vi "monitor -- write section files.vi"(4 "Magn Field (T)":dbl, 6 "temperature":dbl, 10 "Sweep folder path":path=path "C:/Data/GloveBox/Pu-delta-2-20120625/sweep2", 11 "Array":T1[](array[typedef])=[{"delta"=0.0, "gamma"=0.0, "exp"=0.0, "found?"=FALSE, "found"=0.0, "gamma found"=0.0, "init linear"=FALSE, "interpolate"=enum."force", "gamma-factor"=3.5, "slope"=0.0, "update freq?"=FALSE, "update gamma?"=FALSE, "acc factor"=3.5, "linear interpolation state"={"requested size"=20, "Array"=[], "actual number of elements"=0}, "ind"=0.0, "gamma ratio"=0.0, "gamma off limit?"=FALSE, "freq off limit?"=FALSE}, {"delta"=0.0, "gamma"=0.0, "exp"=0.0, "found?"=FALSE, "found"=0.0, "gamma found"=0.0, "init linear"=FALSE, "interpolate"=enum."force", "gamma-factor"=3.5, "slope"=0.0, "update freq?"=FALSE, "update gamma?"=FALSE, "acc factor"=3.5, "linear interpolation state"={"requested size"=20, "Array"=[], "actual number of elements"=0}, "ind"=0.0, "gamma ratio"=0.0, "gamma off limit?"=FALSE, "freq off limit?"=FALSE}, {"delta"=0.0, "gamma"=0.0, "exp"=0.0, "found?"=FALSE, "found"=0.0, "gamma found"=0.0, "init linear"=FALSE, "interpolate"=enum."force", "gamma-factor"=3.5, "slope"=0.0, "update freq?"=FALSE, "update gamma?"=FALSE, "acc factor"=3.5, "linear interpolation state"={"requested size"=20, "Array"=[], "actual number of elements"=0}, "ind"=0.0, "gamma ratio"=0.0, "gamma off limit?"=FALSE, "freq off limit?"=FALSE}, {"delta"=0.0, "gamma"=0.0, "exp"=0.0, "found?"=FALSE, "found"=0.0, "gamma found"=0.0, "init linear"=FALSE, "interpolate"=enum."force", "gamma-factor"=3.5, "slope"=0.0, "update freq?"=FALSE, "update gamma?"=FALSE, "acc factor"=3.5, "linear interpolation state"={"requested size"=20, "Array"=[], "actual number of elements"=0}, "ind"=0.0, "gamma ratio"=0.0, "gamma off limit?"=FALSE, "freq off limit?"=FALSE}, {"delta"=0.0, "gamma"=0.0, "exp"=0.0, "found?"=FALSE, "found"=0.0, "gamma found"=0.0, "init linear"=FALSE, "interpolate"=enum."force", "gamma-factor"=3.5, "slope"=0.0, "update freq?"=FALSE, "update gamma?"=FALSE, "acc factor"=3.5, "linear interpolation state"={"requested size"=20, "Array"=[], "actual number of elements"=0}, "ind"=0.0, "gamma ratio"=0.0, "gamma off limit?"=FALSE, "freq off limit?"=FALSE}, {"delta"=0.0, "gamma"=0.0, "exp"=0.0, "found?"=FALSE, "found"=0.0, "gamma found"=0.0, "init linear"=FALSE, "interpolate"=enum."force", "gamma-factor"=3.5, "slope"=0.0, "update freq?"=FALSE, "update gamma?"=FALSE, "acc factor"=3.5, "linear interpolation state"={"requested size"=20, "Array"=[], "actual number of elements"=0}, "ind"=0.0, "gamma ratio"=0.0, "gamma off limit?"=FALSE, "freq off limit?"=FALSE}, {"delta"=0.0, "gamma"=0.0, "exp"=0.0, "found?"=FALSE, "found"=0.0, "gamma found"=0.0, "init linear"=FALSE, "interpolate"=enum."force", "gamma-factor"=3.5, "slope"=0.0, "update freq?"=FALSE, "update gamma?"=FALSE, "acc factor"=3.5, "linear interpolation state"={"requested size"=20, "Array"=[], "actual number of elements"=0}, "ind"=0.0, "gamma ratio"=0.0, "gamma off limit?"=FALSE, "freq off limit?"=FALSE}, {"delta"=0.0, "gamma"=0.0, "exp"=0.0, "found?"=FALSE, "found"=0.0, "gamma found"=0.0, "init linear"=FALSE, "interpolate"=enum."force", "gamma-factor"=3.5, "slope"=0.0, "update freq?"=FALSE, "update gamma?"=FALSE, "acc factor"=3.5, "linear interpolation state"={"requested size"=20, "Array"=[], "actual number of elements"=0}, "ind"=0.0, "gamma ratio"=0.0, "gamma off limit?"=FALSE, "freq off limit?"=FALSE}, {"delta"=0.0, "gamma"=0.0, "exp"=0.0, "found?"=FALSE, "found"=0.0, "gamma found"=0.0, "init linear"=FALSE, "interpolate"=enum."force", "gamma-factor"=3.5, "slope"=0.0, "update freq?"=FALSE, "update gamma?"=FALSE, "acc factor"=3.5, "linear interpolation state"={"requested size"=20, "Array"=[], "actual number of elements"=0}, "ind"=0.0, "gamma ratio"=0.0, "gamma off limit?"=FALSE, "freq off limit?"=FALSE}, {"delta"=0.0, "gamma"=0.0, "exp"=0.0, "found?"=FALSE, "found"=0.0, "gamma found"=0.0, "init linear"=FALSE, "interpolate"=enum."force", "gamma-factor"=3.5, "slope"=0.0, "update freq?"=FALSE, "update gamma?"=FALSE, "acc factor"=3.5, "linear interpolation state"={"requested size"=20, "Array"=[], "actual number of elements"=0}, "ind"=0.0, "gamma ratio"=0.0, "gamma off limit?"=FALSE, "freq off limit?"=FALSE}, {"delta"=0.0, "gamma"=0.0, "exp"=0.0, "found?"=FALSE, "found"=0.0, "gamma found"=0.0, "init linear"=FALSE, "interpolate"=enum."force", "gamma-factor"=3.5, "slope"=0.0, "update freq?"=FALSE, "update gamma?"=FALSE, "acc factor"=3.5, "linear interpolation state"={"requested size"=20, "Array"=[], "actual number of elements"=0}, "ind"=0.0, "gamma ratio"=0.0, "gamma off limit?"=FALSE, "freq off limit?"=FALSE}, {"delta"=0.0, "gamma"=0.0, "exp"=0.0, "found?"=FALSE, "found"=0.0, "gamma found"=0.0, "init linear"=FALSE, "interpolate"=enum."force", "gamma-factor"=3.5, "slope"=0.0, "update freq?"=FALSE, "update gamma?"=FALSE, "acc factor"=3.5, "linear interpolation state"={"requested size"=20, "Array"=[], "actual number of elements"=0}, "ind"=0.0, "gamma ratio"=0.0, "gamma off limit?"=FALSE, "freq off limit?"=FALSE}, {"delta"=0.0, "gamma"=0.0, "exp"=0.0, "found?"=FALSE, "found"=0.0, "gamma found"=0.0, "init linear"=FALSE, "interpolate"=enum."force", "gamma-factor"=3.5, "slope"=0.0, "update freq?"=FALSE, "update gamma?"=FALSE, "acc factor"=3.5, "linear interpolation state"={"requested size"=20, "Array"=[], "actual number of elements"=0}, "ind"=0.0, "gamma ratio"=0.0, "gamma off limit?"=FALSE, "freq off limit?"=FALSE}, {"delta"=0.0, "gamma"=0.0, "exp"=0.0, "found?"=FALSE, "found"=0.0, "gamma found"=0.0, "init linear"=FALSE, "interpolate"=enum."force", "gamma-factor"=3.5, "slope"=0.0, "update freq?"=FALSE, "update gamma?"=FALSE, "acc factor"=3.5, "linear interpolation state"={"requested size"=20, "Array"=[], "actual number of elements"=0}, "ind"=0.0, "gamma ratio"=0.0, "gamma off limit?"=FALSE, "freq off limit?"=FALSE}, {"delta"=0.0, "gamma"=0.0, "exp"=0.0, "found?"=FALSE, "found"=0.0, "gamma found"=0.0, "init linear"=FALSE, "interpolate"=enum."force", "gamma-factor"=3.5, "slope"=0.0, "update freq?"=FALSE, "update gamma?"=FALSE, "acc factor"=3.5, "linear interpolation state"={"requested size"=20, "Array"=[], "actual number of elements"=0}, "ind"=0.0, "gamma ratio"=0.0, "gamma off limit?"=FALSE, "freq off limit?"=FALSE}, {"delta"=0.0, "gamma"=0.0, "exp"=0.0, "found?"=FALSE, "found"=0.0, "gamma found"=0.0, "init linear"=FALSE, "interpolate"=enum."force", "gamma-factor"=3.5, "slope"=0.0, "update freq?"=FALSE, "update gamma?"=FALSE, "acc factor"=3.5, "linear interpolation state"={"requested size"=20, "Array"=[], "actual number of elements"=0}, "ind"=0.0, "gamma ratio"=0.0, "gamma off limit?"=FALSE, "freq off limit?"=FALSE}, {"delta"=0.0, "gamma"=0.0, "exp"=0.0, "found?"=FALSE, "found"=0.0, "gamma found"=0.0, "init linear"=FALSE, "interpolate"=enum."force", "gamma-factor"=3.5, "slope"=0.0, "update freq?"=FALSE, "update gamma?"=FALSE, "acc factor"=3.5, "linear interpolation state"={"requested size"=20, "Array"=[], "actual number of elements"=0}, "ind"=0.0, "gamma ratio"=0.0, "gamma off limit?"=FALSE, "freq off limit?"=FALSE}, {"delta"=0.0, "gamma"=0.0, "exp"=0.0, "found?"=FALSE, "found"=0.0, "gamma found"=0.0, "init linear"=FALSE, "interpolate"=enum."force", "gamma-factor"=3.5, "slope"=0.0, "update freq?"=FALSE, "update gamma?"=FALSE, "acc factor"=3.5, "linear interpolation state"={"requested size"=20, "Array"=[], "actual number of elements"=0}, "ind"=0.0, "gamma ratio"=0.0, "gamma off limit?"=FALSE, "freq off limit?"=FALSE}, {"delta"=0.0, "gamma"=0.0, "exp"=0.0, "found?"=FALSE, "found"=0.0, "gamma found"=0.0, "init linear"=FALSE, "interpolate"=enum."force", "gamma-factor"=3.5, "slope"=0.0, "update freq?"=FALSE, "update gamma?"=FALSE, "acc factor"=3.5, "linear interpolation state"={"requested size"=20, "Array"=[], "actual number of elements"=0}, "ind"=0.0, "gamma ratio"=0.0, "gamma off limit?"=FALSE, "freq off limit?"=FALSE}, {"delta"=0.0, "gamma"=0.0, "exp"=0.0, "found?"=FALSE, "found"=0.0, "gamma found"=0.0, "init linear"=FALSE, "interpolate"=enum."force", "gamma-factor"=3.5, "slope"=0.0, "update freq?"=FALSE, "update gamma?"=FALSE, "acc factor"=3.5, "linear interpolation state"={"requested size"=20, "Array"=[], "actual number of elements"=0}, "ind"=0.0, "gamma ratio"=0.0, "gamma off limit?"=FALSE, "freq off limit?"=FALSE}, {"delta"=0.0, "gamma"=0.0, "exp"=0.0, "found?"=FALSE, "found"=0.0, "gamma found"=0.0, "init linear"=FALSE, "interpolate"=enum."force", "gamma-factor"=3.5, "slope"=0.0, "update freq?"=FALSE, "update gamma?"=FALSE, "acc factor"=3.5, "linear interpolation state"={"requested size"=20, "Array"=[], "actual number of elements"=0}, "ind"=0.0, "gamma ratio"=0.0, "gamma off limit?"=FALSE, "freq off limit?"=FALSE}, {"delta"=0.0, "gamma"=0.0, "exp"=0.0, "found?"=FALSE, "found"=0.0, "gamma found"=0.0, "init linear"=FALSE, "interpolate"=enum."force", "gamma-factor"=3.5, "slope"=0.0, "update freq?"=FALSE, "update gamma?"=FALSE, "acc factor"=3.5, "linear interpolation state"={"requested size"=20, "Array"=[], "actual number of elements"=0}, "ind"=0.0, "gamma ratio"=0.0, "gamma off limit?"=FALSE, "freq off limit?"=FALSE}, {"delta"=0.0, "gamma"=0.0, "exp"=0.0, "found?"=FALSE, "found"=0.0, "gamma found"=0.0, "init linear"=FALSE, "interpolate"=enum."force", "gamma-factor"=3.5, "slope"=0.0, "update freq?"=FALSE, "update gamma?"=FALSE, "acc factor"=3.5, "linear interpolation state"={"requested size"=20, "Array"=[], "actual number of elements"=0}, "ind"=0.0, "gamma ratio"=0.0, "gamma off limit?"=FALSE, "freq off limit?"=FALSE}, {"delta"=0.0, "gamma"=0.0, "exp"=0.0, "found?"=FALSE, "found"=0.0, "gamma found"=0.0, "init linear"=FALSE, "interpolate"=enum."force", "gamma-factor"=3.5, "slope"=0.0, "update freq?"=FALSE, "update gamma?"=FALSE, "acc factor"=3.5, "linear interpolation state"={"requested size"=20, "Array"=[], "actual number of elements"=0}, "ind"=0.0, "gamma ratio"=0.0, "gamma off limit?"=FALSE, "freq off limit?"=FALSE}, {"delta"=0.0, "gamma"=0.0, "exp"=0.0, "found?"=FALSE, "found"=0.0, "gamma found"=0.0, "init linear"=FALSE, "interpolate"=enum."force", "gamma-factor"=3.5, "slope"=0.0, "update freq?"=FALSE, "update gamma?"=FALSE, "acc factor"=3.5, "linear interpolation state"={"requested size"=20, "Array"=[], "actual number of elements"=0}, "ind"=0.0, "gamma ratio"=0.0, "gamma off limit?"=FALSE, "freq off limit?"=FALSE}, {"delta"=0.0, "gamma"=0.0, "exp"=0.0, "found?"=FALSE, "found"=0.0, "gamma found"=0.0, "init linear"=FALSE, "interpolate"=enum."force", "gamma-factor"=3.5, "slope"=0.0, "update freq?"=FALSE, "update gamma?"=FALSE, "acc factor"=3.5, "linear interpolation state"={"requested size"=20, "Array"=[], "actual number of elements"=0}, "ind"=0.0, "gamma ratio"=0.0, "gamma off limit?"=FALSE, "freq off limit?"=FALSE}, {"delta"=0.0, "gamma"=0.0, "exp"=0.0, "found?"=FALSE, "found"=0.0, "gamma found"=0.0, "init linear"=FALSE, "interpolate"=enum."force", "gamma-factor"=3.5, "slope"=0.0, "update freq?"=FALSE, "update gamma?"=FALSE, "acc factor"=3.5, "linear interpolation state"={"requested size"=20, "Array"=[], "actual number of elements"=0}, "ind"=0.0, "gamma ratio"=0.0, "gamma off limit?"=FALSE, "freq off limit?"=FALSE}, {"delta"=0.0, "gamma"=0.0, "exp"=0.0, "found?"=FALSE, "found"=0.0, "gamma found"=0.0, "init linear"=FALSE, "interpolate"=enum."force", "gamma-factor"=3.5, "slope"=0.0, "update freq?"=FALSE, "update gamma?"=FALSE, "acc factor"=3.5, "linear interpolation state"={"requested size"=20, "Array"=[], "actual number of elements"=0}, "ind"=0.0, "gamma ratio"=0.0, "gamma off limit?"=FALSE, "freq off limit?"=FALSE}, {"delta"=0.0, "gamma"=0.0, "exp"=0.0, "found?"=FALSE, "found"=0.0, "gamma found"=0.0, "init linear"=FALSE, "interpolate"=enum."force", "gamma-factor"=3.5, "slope"=0.0, "update freq?"=FALSE, "update gamma?"=FALSE, "acc factor"=3.5, "linear interpolation state"={"requested size"=20, "Array"=[], "actual number of elements"=0}, "ind"=0.0, "gamma ratio"=0.0, "gamma off limit?"=FALSE, "freq off limit?"=FALSE}, {"delta"=0.0, "gamma"=0.0, "exp"=0.0, "found?"=FALSE, "found"=0.0, "gamma found"=0.0, "init linear"=FALSE, "interpolate"=enum."force", "gamma-factor"=3.5, "slope"=0.0, "update freq?"=FALSE, "update gamma?"=FALSE, "acc factor"=3.5, "linear interpolation state"={"requested size"=20, "Array"=[], "actual number of elements"=0}, "ind"=0.0, "gamma ratio"=0.0, "gamma off limit?"=FALSE, "freq off limit?"=FALSE}, {"delta"=0.0, "gamma"=0.0, "exp"=0.0, "found?"=FALSE, "found"=0.0, "gamma found"=0.0, "init linear"=FALSE, "interpolate"=enum."force", "gamma-factor"=3.5, "slope"=0.0, "update freq?"=FALSE, "update gamma?"=FALSE, "acc factor"=3.5, "linear interpolation state"={"requested size"=20, "Array"=[], "actual number of elements"=0}, "ind"=0.0, "gamma ratio"=0.0, "gamma off limit?"=FALSE, "freq off limit?"=FALSE}, {"delta"=0.0, "gamma"=0.0, "exp"=0.0, "found?"=FALSE, "found"=0.0, "gamma found"=0.0, "init linear"=FALSE, "interpolate"=enum."force", "gamma-factor"=3.5, "slope"=0.0, "update freq?"=FALSE, "update gamma?"=FALSE, "acc factor"=3.5, "linear interpolation state"={"requested size"=20, "Array"=[], "actual number of elements"=0}, "ind"=0.0, "gamma ratio"=0.0, "gamma off limit?"=FALSE, "freq off limit?"=FALSE}, {"delta"=0.0, "gamma"=0.0, "exp"=0.0, "found?"=FALSE, "found"=0.0, "gamma found"=0.0, "init linear"=FALSE, "interpolate"=enum."force", "gamma-factor"=3.5, "slope"=0.0, "update freq?"=FALSE, "update gamma?"=FALSE, "acc factor"=3.5, "linear interpolation state"={"requested size"=20, "Array"=[], "actual number of elements"=0}, "ind"=0.0, "gamma ratio"=0.0, "gamma off limit?"=FALSE, "freq off limit?"=FALSE}]) -> ()   [LabVIEW 2015]
uses:
  peak monitor ctl - V2.ctl
  interpolation state - real.ctl
  lorentzian.ctl
  circle corners.ctl
  ctl -- name dispatcher -- action.ctl
  next chunk read-write PID -- action.ctl
  file -- read-write control.ctl
  array -- find index - real.vi
  array -- interpolate -- i.vi
  Q -- check range -- i -- real.vi
  Q - not nan -- real.vi
  <vilib>/Utility/libraryn.llb/Check if File or Folder Exists.vi
  file -- read list of lines.vi
  parse -- find first line.vi
  parse -- get list of matches -- numbers.vi
  <vilib>/Utility/file.llb/Write To Spreadsheet File.vi
  <vilib>/Utility/file.llb/Write To Spreadsheet File (string).vi
  <vilib>/gmath/function.llb/Binomial Coefficient.vi
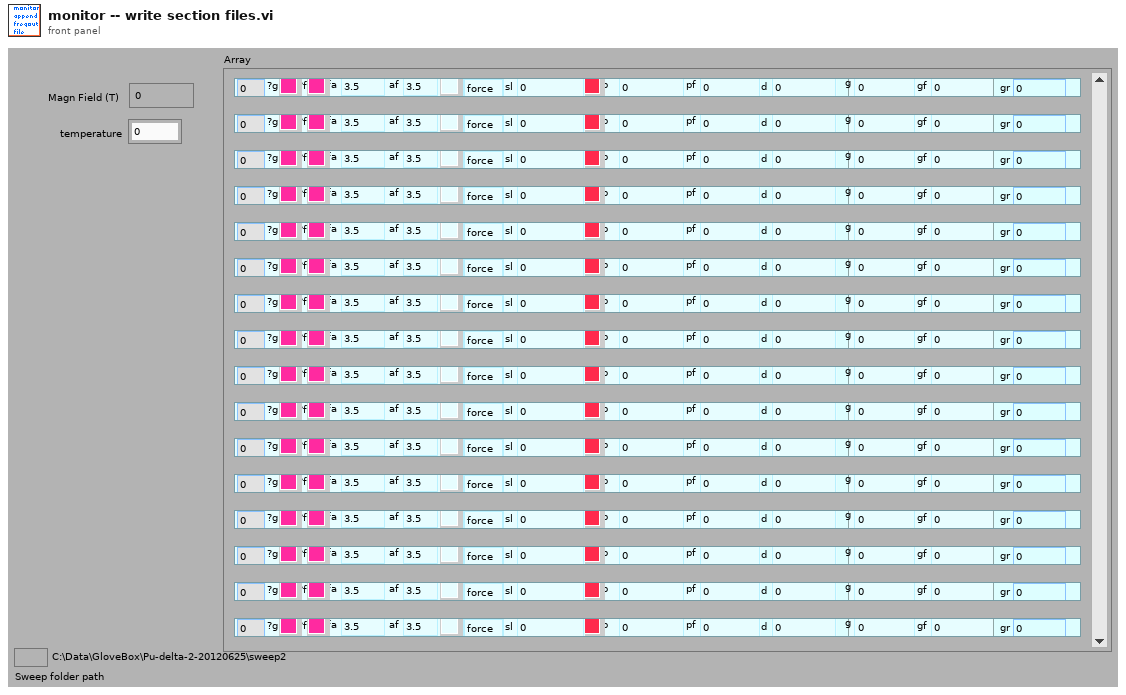
[diagram p1: front panel]
types:
  T1 = typedef "peak monitor ctl - V2.ctl" = cluster{"delta":dbl, "gamma":dbl, "exp":dbl, "found?":bool, "found":dbl, "gamma found":dbl, "init linear":bool, "interpolate":enum16{"line", "force"}, "gamma-factor":dbl, "slope":dbl, "update freq?":bool, "update gamma?":bool, "acc factor":dbl, "linear interpolation state":T2, "ind":dbl, "gamma ratio":dbl, "gamma off limit?":bool, "freq off limit?":bool}
  T2 = typedef "interpolation state - real.ctl" = cluster{"requested size":i32, "Array":dbl[], "actual number of elements":i32}
  T3 = typedef "ctl -- name dispatcher -- action.ctl" = enum16{"peak frequency", "peak frequency DUMP", "peak gamma DUMP", "peak gamma", "peak frequency TEST", "peak gamma TEST", "ultrasonic power", "time in gamma", "set temperature ", "set temperature timer", "peak default gamma", "last scan file", "peak freq gamma TEST", "peak NAMES", "errors", "P_I_D", "P", "I", "D", "power vs time", "power vs time TIMER", "void", "power log", "set temperature - SINE", "itc ltc log", "peak - time in gamma"}
  T4 = typedef "lorentzian.ctl" = cluster{"Amplitude":dbl, "omega(0)":dbl, "Gamma":dbl, "phase":dbl, "Q":dbl, "Norm  Ampl":dbl, "z (inf)":cdb, "4corners":T5}
  T5 = typedef "circle corners.ctl" = cluster{"z (-pi/2)":cdb, "z(inf)":cdb, "z (pi/2)":cdb, "z center":cdb, "z(0)":cdb, "radius":dbl}
  T6 = typedef "next chunk read-write PID -- action.ctl" = enum16{"read", "interpolate", "append col", "write", "write PID col", "append PID col", "interpolate - bezier"}
  T7 = typedef "file -- read-write control.ctl" = enum16{"read", "write all", "append one line"}
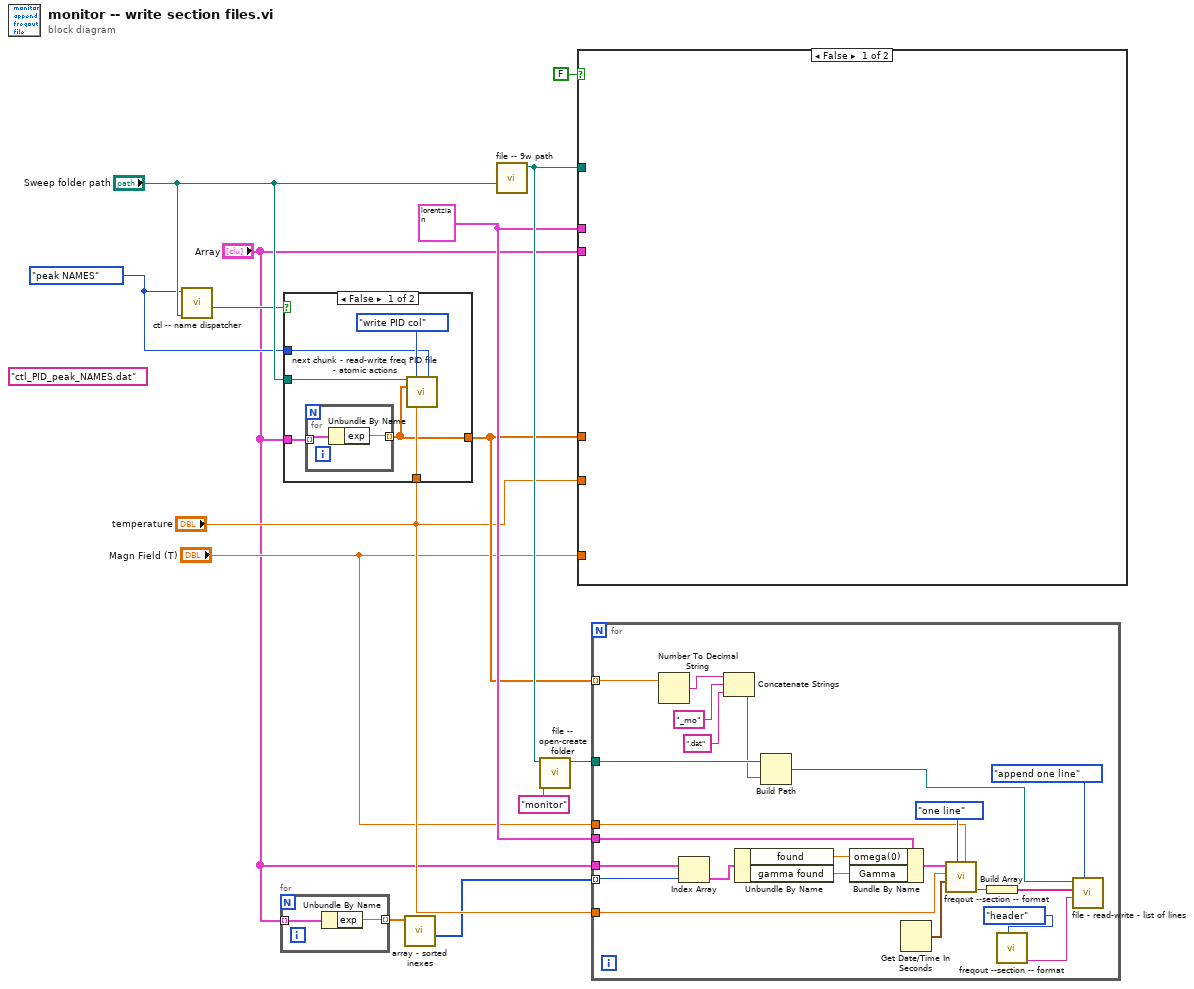
[diagram p0: block diagram]
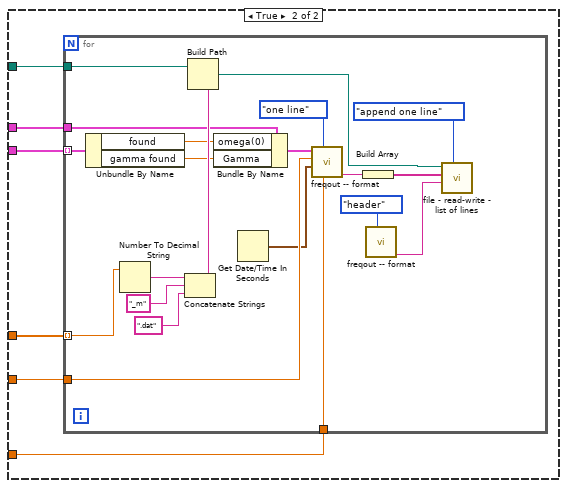
[diagram p2: hidden frame]
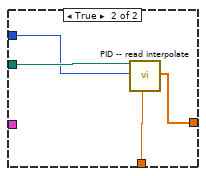
[diagram p3: hidden frame]
diagram:
  w6 = ctl_--_name_dispatcher_--_action."peak NAMES" ("ctl kind")
  w12 = T4 {"Amplitude"=0.0, "omega(0)"=0.0, "Gamma"=0.0, "phase"=0.0, "Q"=0.0, "Norm  Ampl"=0.0, "z (inf)"=0.0+0.0i, "4corners"={"z (-pi/2)"=0.0+0.0i, "z(inf)"=0.0+0.0i, "z (pi/2)"=0.0+0.0i, "z center"=0.0+0.0i, "z(0)"=0.0+0.0i, "radius"=0.0}} ("lorentzian")
  (unwired) "ctl_PID_peak_NAMES.dat" ("freq PID file IN")
  n1 = call "ctl -- name dispatcher.vi"("sweep folder path"="Sweep folder path", "ctl name dispatch"=w6) -> ("file or folder exists?"=w7:bool)  [unwired: 7 in, 2 out]
  n2 = for {
    tunnel: "Array" -> [w16] mode=indexing
    tunnel: [w15] -> w2 mode=indexing
    n3 = Unbundle By Name(w16) -> ("exp"=w15:dbl)
  }
  n4 = case shown="False" w7 {
    tunnel: "Sweep folder path" -> [w21 w26]
    tunnel: [w18 w28] -> w10
    tunnel: "temperature" -> [w19 w27]
    tunnel: w6 -> [w20 w25]
    tunnel: "Array" -> [w17 _]
    frame False {
      n5 = for {
        tunnel: w17 -> [w24] mode=indexing
        tunnel: [w23] -> w18 mode=indexing
        n6 = Unbundle By Name(w24) -> ("exp"=w23:dbl)
      }
      n7 = call "next chunk - read-write freq PID file - atomic actions .vi"("sweep folder path"=w21, "PID action"=next_chunk_read-write_PID_--_action."write PID col", "ctl kind OUT"=w20, "PID freq IN"=w18, "temperature"=w19) -> ()  [unwired: 6 in, 5 out]
    }
    frame True {
      n8 = call "PID -- read interpolate.vi"("sweep folder path"=w26, "ctl PID file IN"=w25, "temperature"=w27) -> ("PID freq"=w28:dbl[])  [unwired: 11 in, 5 out]
    }
  }
  n9 = call "array - sorted inexes.vi"("x"=w2) -> ("index array"=w1:i32[])  [unwired: 9 in, 1 out]
  n10 = call "file -- 9w path.vi"("sweep folder"="Sweep folder path") -> ("9w path"=w13:path)  [unwired: 10 in]
  n11 = call "file -- open-create folder.vi"("folder name"="monitor" ("name or relative path"), "base path"=w13) -> ("folder path out"=w11:path)  [unwired: 9 in]
  n12 = case shown="False" FALSE {
    tunnel: w13 -> [_ w34]
    tunnel: w12 -> [_ w33]
    tunnel: w10 -> [_ w32]
    tunnel: "temperature" -> [_ w31]
    tunnel: "Array" -> [_ w30]
    tunnel: "Magn Field (T)" -> [_ w29]
    frame False {
    }
    frame True {
      n13 = for {
        tunnel: w30 -> [w49] mode=indexing
        tunnel: w34 -> [w55]
        tunnel: w32 -> [w54] mode=indexing
        tunnel: w33 -> [w48]
        tunnel: w31 -> [w44]
        tunnel: w29 -> [w41]
        n14 = Unbundle By Name(w49) -> ("found"=w46:dbl, "gamma found"=w47:dbl)
        n15 = Number To Decimal String(number=w54) -> (decimal integer string=w53:string)  [unwired: 1 in]
        n16 = Concatenate Strings(w53, "_m" ("string"), ".dat" ("string")) -> (w51:string)
        n17 = Build Path(base path=w55, name or relative path=w51) -> (appended path=w35:path)
        n18 = Bundle By Name(cluster=w48, "omega(0)"=w46, "Gamma"=w47) -> (w45:T4)
        n19 = Get Date/Time In Seconds() -> (seconds since 1Jan1904=w43:timestamp)
        n20 = call "freqout -- format.vi"("Magn Field (T)"=w41, "freqout action"=enum16{"header", "one line", "one"}."one line", "timestamp"=w43, "temperature"=w44, "lorentzian"=w45) -> ("output string"=w38:string)  [unwired: 6 in]
        n21 = Build Array(w38) -> (w37:string[])
        n22 = call "freqout -- format.vi"("freqout action"=enum16{"header", "one line", "one"}."header") -> ("output string"=w36:string)  [unwired: 10 in]
        n23 = call "file - read-write - list of lines.vi"("read/write control"=file_--_read-write_control."append one line", "header"=w36, "list of lines IN"=w37, "file path"=w35) -> ()  [unwired: 6 in, 2 out]
      }
    }
  }
  n24 = for {
    tunnel: "Array" -> [w58]
    tunnel: w11 -> [w78]
    tunnel: w10 -> [w77] mode=indexing
    tunnel: w12 -> [w72]
    tunnel: "temperature" -> [w68]
    tunnel: "Magn Field (T)" -> [w65]
    tunnel: w1 -> [w57] mode=indexing
    n25 = Number To Decimal String(number=w77) -> (decimal integer string=w76:string)  [unwired: 1 in]
    n26 = Index Array(array=w58, index=w57) -> (element=w56:T1)
    n27 = Concatenate Strings(w76, "_mo" ("string"), ".dat" ("string")) -> (w74:string)
    n28 = Unbundle By Name(w56) -> ("found"=w70:dbl, "gamma found"=w71:dbl)
    n29 = Build Path(base path=w78, name or relative path=w74) -> (appended path=w61:path)
    n30 = Bundle By Name(cluster=w72, "omega(0)"=w70, "Gamma"=w71) -> (w69:T4)
    n31 = Get Date/Time In Seconds() -> (seconds since 1Jan1904=w67:timestamp)
    n32 = call "freqout --section -- format.vi"("Magn Field (T)"=w65, "freqout action"=enum16{"header", "one line", "one"}."one line", "timestamp"=w67, "temperature"=w68, "lorentzian"=w69) -> ("output string"=w64:string)  [unwired: 6 in]
    n33 = Build Array(w64) -> (w59:string[])
    n34 = call "freqout --section -- format.vi"("freqout action"=enum16{"header", "one line", "one"}."header") -> ("output string"=w60:string)  [unwired: 10 in]
    n35 = call "file - read-write - list of lines.vi"("read/write control"=file_--_read-write_control."append one line", "header"=w60, "list of lines IN"=w59, "file path"=w61) -> ()  [unwired: 6 in, 2 out]
  }
